vi "SeCrTs-Data Transfer Loop DD.vi"(9 "Data FIFO Ref":T1) -> ()   [LabVIEW 2022 SP3]
uses:
  RT Controls/SeCrTs-Data FIFO.ctl
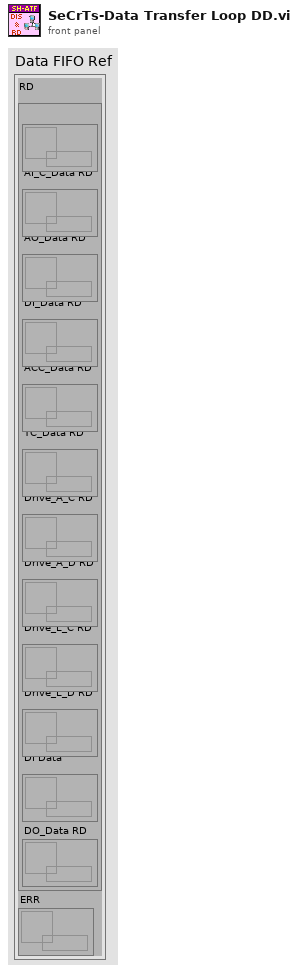
[diagram p1: front panel]
types:
  T1 = typedef "SeCrTs-Data FIFO.ctl" = cluster{"RD":cluster{"AI_V_Data RD":refnum<queue>, "AI_C_Data RD":refnum<queue>, "AO_Data RD":refnum<queue>, "DI_Data RD":refnum<queue>, "ACC_Data RD":refnum<queue>, "TC_Data RD":refnum<queue>, "Drive_A_C RD":refnum<queue>, "Drive_A_D RD":refnum<queue>, "Drive_L_C RD":refnum<queue>, "Drive_L_D RD":refnum<queue>, "DI Data":refnum<queue>, "DO_Data RD":refnum<queue>}, "ERR":refnum<queue>}
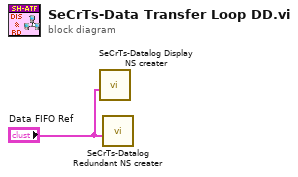
[diagram p0: block diagram]
diagram:
  n1 = call "SeCrTs-Datalog Display NS creater.vi"("Data FIFO Ref"="Data FIFO Ref") -> ()  [unwired: 11 in]
  n2 = call "SeCrTs-Datalog Redundant NS creater.vi"("Data FIFO Ref"="Data FIFO Ref") -> ()  [unwired: 11 in]
